vi "add assembly.vi"(6 "size (bytes)":u32=32, 7 "name":string, 8 "error in":errorcluster, 9 "Type":T1, 10 "instance ID":u32=100, 11 "EthernetIP configuration in":refnum<class "EthernetIP configuration.lvclass">) -> (0 "error out":errorcluster, 3 "EthernetIP configuration out":refnum<class "EthernetIP configuration.lvclass">)   [LabVIEW 2013, in "EthernetIP configuration.lvclass"]
uses:
  EthernetIP configuration.lvclass
  assembly type.ctl
  EthernetIP configuration.lvclass/EthernetIP configuration.ctl
  assembly definition.ctl
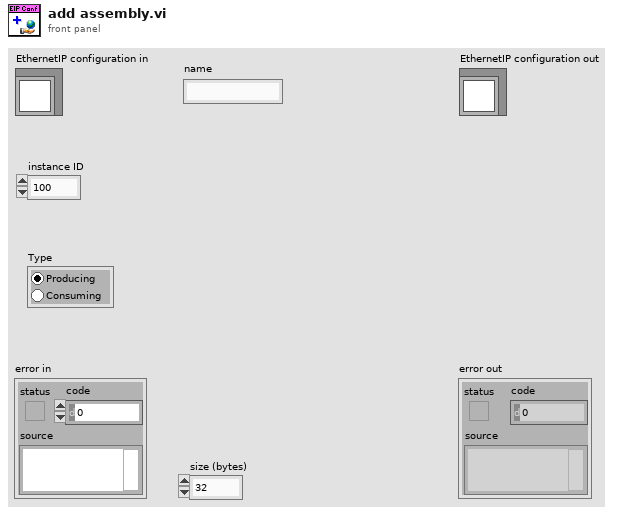
[diagram p1: front panel]
types:
  T1 = typedef "EthernetIP configuration.lvclass/assembly type.ctl" = enum32{"Producing", "Consuming"}
  T2 = typedef "EthernetIP configuration.lvclass/assembly definition.ctl" = cluster{"name":string, "Instance ID":u32, "Type":T1, "Size (bytes)":u32}
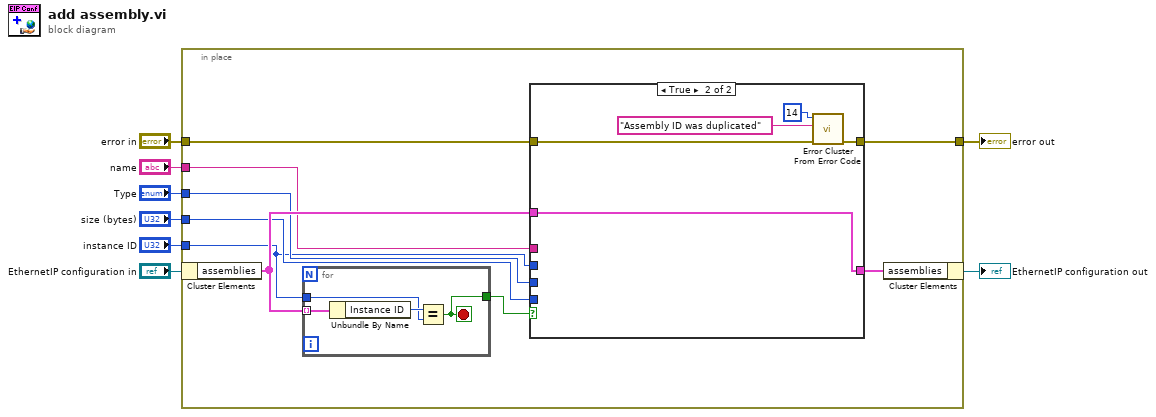
[diagram p0: block diagram]
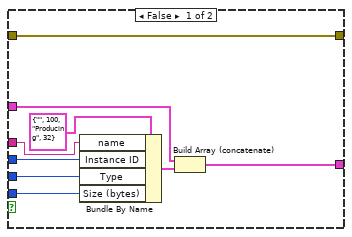
[diagram p2: hidden frame]
diagram:
  n1 = in-place {
    in-place-border: "instance ID" -> [w10]
    in-place-border: "error in" -> [w14]
    in-place-border: [w13] -> w4
    in-place-border: "size (bytes)" -> [w12]
    in-place-border: "Type" -> [w11]
    in-place-border: "name" -> [w9]
    n2 = in-place-cluster #1("EthernetIP configuration in") -> ("assemblies"=w15:T2[])
    n3 = for {
      tunnel: w15 -> [w35] mode=indexing
      tunnel: w10 -> [w33]
      tunnel: [w32] -> w17
      stop <- w32 stop-if-true
      n4 = Unbundle By Name(w35) -> ("Instance ID"=w34:u32)
      n5 = Equal?(x=w34, y=w33) -> (x = y?=w32:bool)
    }
    n6 = case shown="True" w17 {
      tunnel: [w24 w31] -> w16
      tunnel: w15 -> [w25 w31]
      tunnel: w14 -> [w26 w28]
      tunnel: [w26 w27] -> w13
      tunnel: w12 -> [w22 _]
      tunnel: w11 -> [w21 _]
      tunnel: w10 -> [w20 _]
      tunnel: w9 -> [w19 _]
      frame False {
        n7 = Bundle By Name(cluster=T2 {"name"="", "Instance ID"=100, "Type"=enum."Producing", "Size (bytes)"=32} ("assembly definition"), "name"=w19, "Instance ID"=w20, "Type"=w21, "Size (bytes)"=w22) -> (w18:T2)
        n8 = Build Array (concatenate)(w25, w18) -> (w24:T2[])
      }
      frame True {
        n9 = call <vilib>:"Error Cluster From Error Code.vi"("error in (no error)"=w28, "error message (\"\")"="Assembly ID was duplicated" ("error message (\"\")"), "error code (0)"=14) -> ("error out"=w27:errorcluster)  [unwired: 6 in]
      }
    }
    n10 = in-place-cluster #1("assemblies"=w16) -> (→"EthernetIP configuration out":refnum<class "EthernetIP configuration.lvclass">)
  }
  "error out" <- w4
